vi "Modules - Test Panel.vi"(8 "error in":errorcluster) -> (0 "error out":errorcluster)   [LabVIEW 2019]
uses:
  Controls/Station - Test Type.ctl
  Controls/Test Panel - State.ctl
  Controls/eFGV States.ctl
  Controls/FGV States.ctl
  Controls/Test Panel - Data Structure.ctl
  <vilib>/Utility/miscctls.llb/LVRowAndColumnTypeDef.ctl
panel:
  in  "Add Station":bool
  in  "Test Type":T1 items=["Please Select", "Triaxial Shear", "Triaxial UU", "Shearbox", "Permeability", "Consolidation (Stepped Loading)/Swelling", "Saturation (Incremental)", "User Defined", "UCT", "Isotropic Consolidation", "Swelling Pressure"]
  in  "Data Save":bool
  out "Job Description :":string
  out "Job No :":string
  out "Sample No :":string
  in  "Add Test":bool
  in  "Sample":bool
  in  "Tab":enum32{"Test Stages"}(tab)
  out "Table":string[][](table)
  in  "Next Stage":bool caption="Go to next Stage \nautomatically"
  in  "Run":bool
  in  "Remove":bool
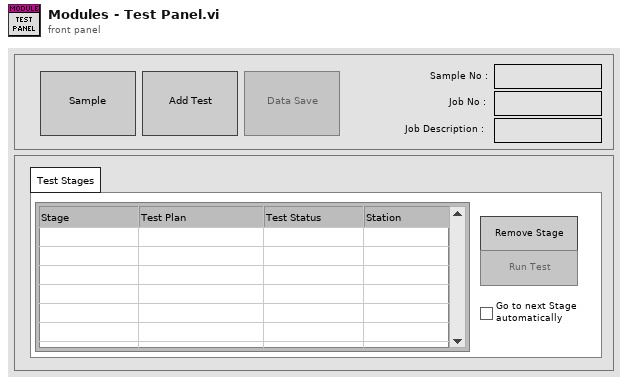
[diagram p1: front panel]
types:
  T1 = typedef "Station - Test Type.ctl" = u16
  T2 = typedef "Test Panel - State.ctl" = enum16{"Init", "Idle", "Load", "Run", "Add Test", "Highlight", "Up", "Down", "Manual", "Clear Data", "Save List", "Load List", "Change Station", "Close"}
  T3 = typedef "Test Panel - Data Structure.ctl" = cluster{"Station":string, "Sample ID":string, "Job No":string, "Job Description":string, "Filename":string, "Test Type":T1, "Speciment No":string, "Depth":string, "Height":string, "Diameter/Length":string, "Weight":string, "Test Parameter":string, "Station[]":string[], "Edit Pos":T4, "Edit Pos Prev":T4, "Area":string, "Path":string}
  T4 = typedef "LVRowAndColumnTypeDef.ctl" = cluster{"Row":i32, "Column":i32}
  T5 = enum8{"Enabled", "Disabled", "Disabled and Grayed Out"}
  T6 = typedef "FGV States.ctl" = enum16{"Read", "Write"}
  T7 = enum32{"Invalid", "Standard", "Closed", "Hidden", "Minimized", "Maximized"}
  T8 = typedef "eFGV States.ctl" = enum16{"Init", "Read", "Write", "Exit"}
  T9 = cluster{"Sample No":string, "Job No":string, "Job Desc":string, "Save":bool, "Speciment No":string, "Depth":string, "Height":string, "Diameter/Length":string, "Weight":string, "JobNo []":string[], "JobID []":string[], "JobDesc []":string[], "Speciment []":string[], "attribute":string}
  T10 = cluster{"Station Name":string, "Key Value":string[], "Key Names":string[]}[]
  T11 = cluster{"Station Name":string, "Key Value":string[], "Key Names":string[]}
  T12 = enum32{"invalid app kind", "Development System", "Run Time System", "Student Edition", "Embedded LabVIEW", "Evaluation", "Custom"}
  T13 = cluster{"TestPlan Section":string, "Key Value":string[]}[]
  T14 = cluster{"TestPlan Section":string, "Key Value":string[]}
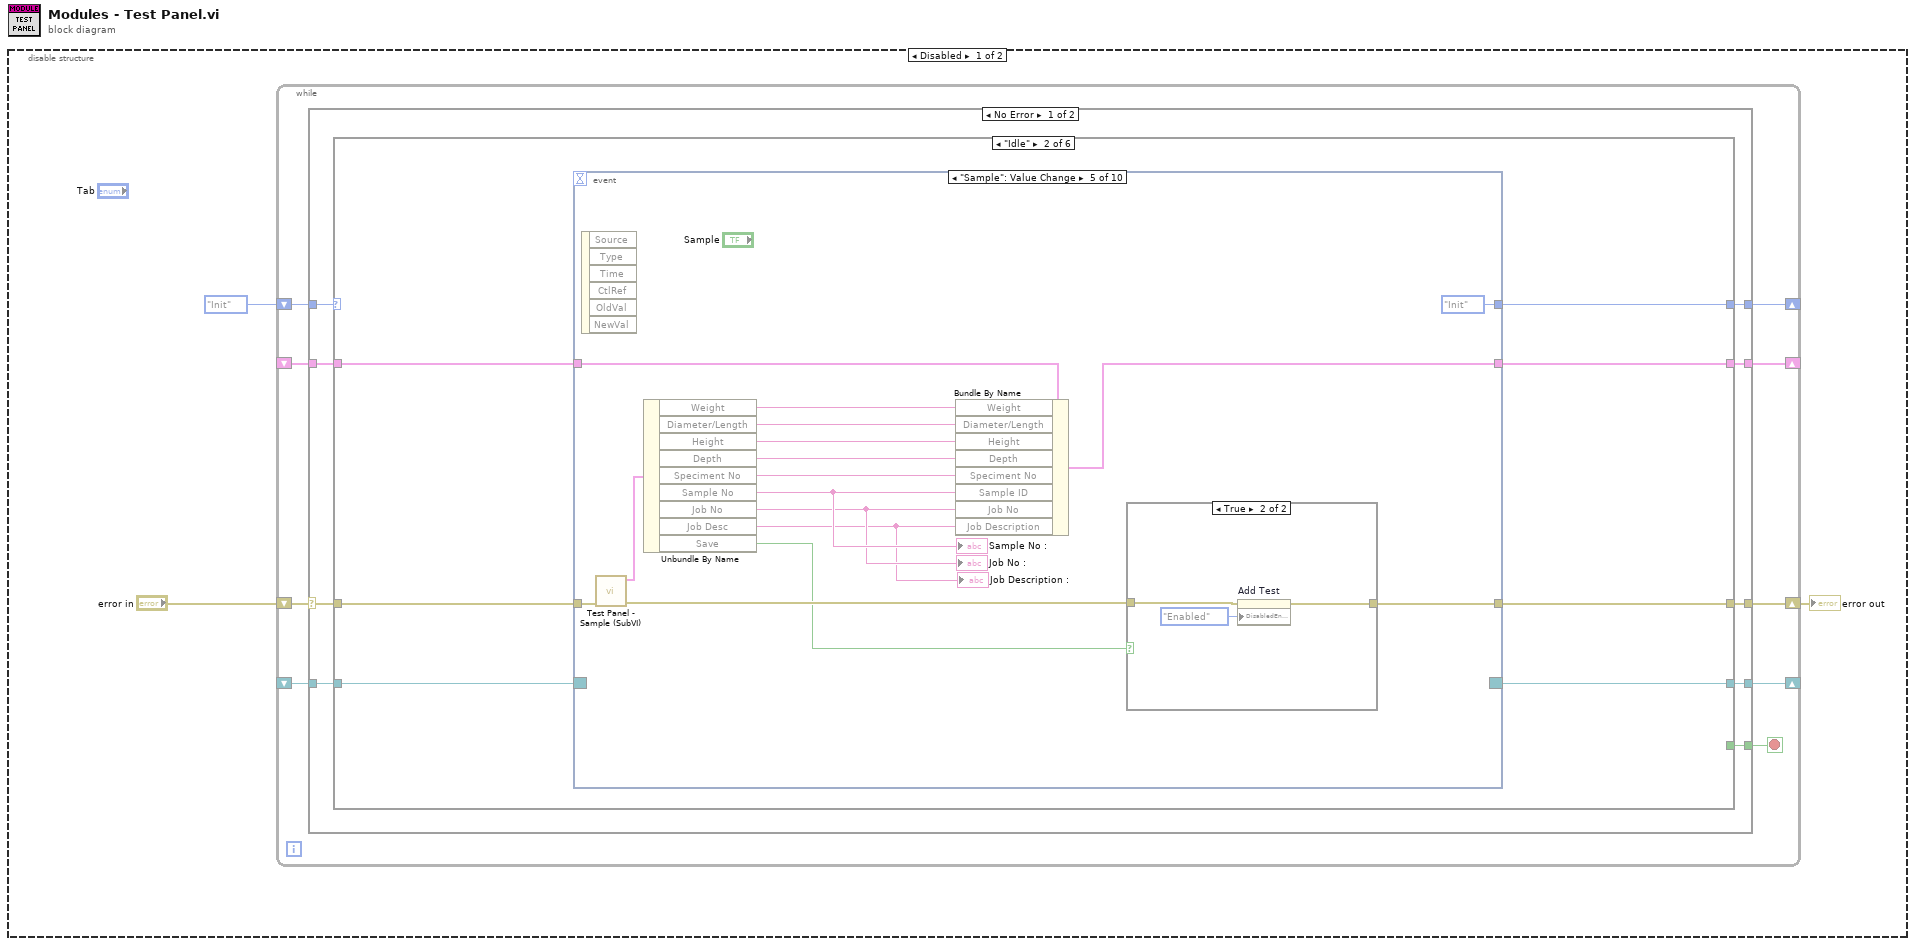
[diagram p0: block diagram]
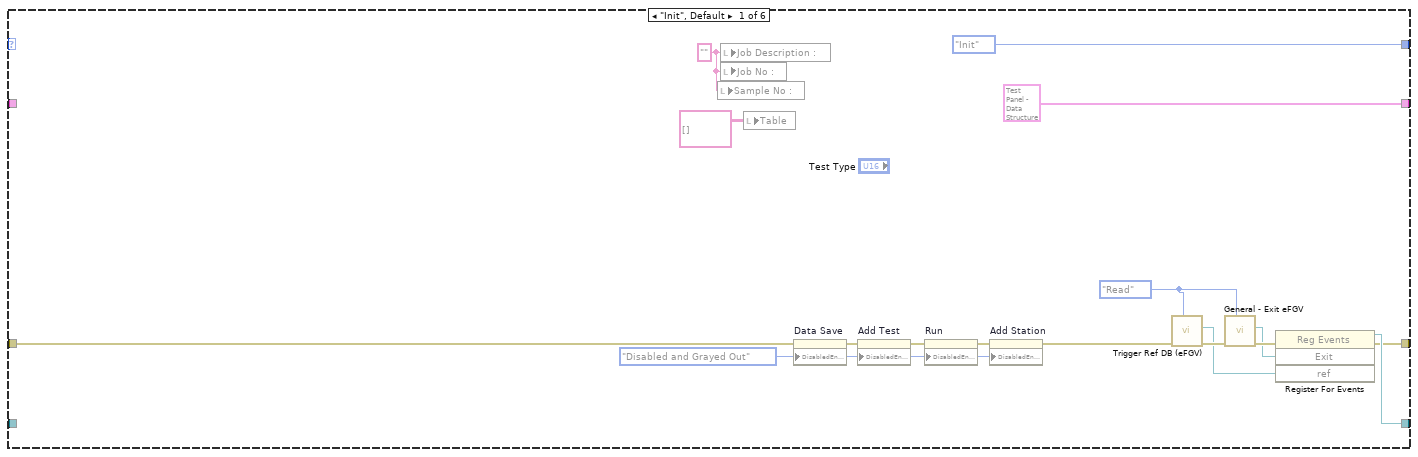
[diagram p2: hidden frame]
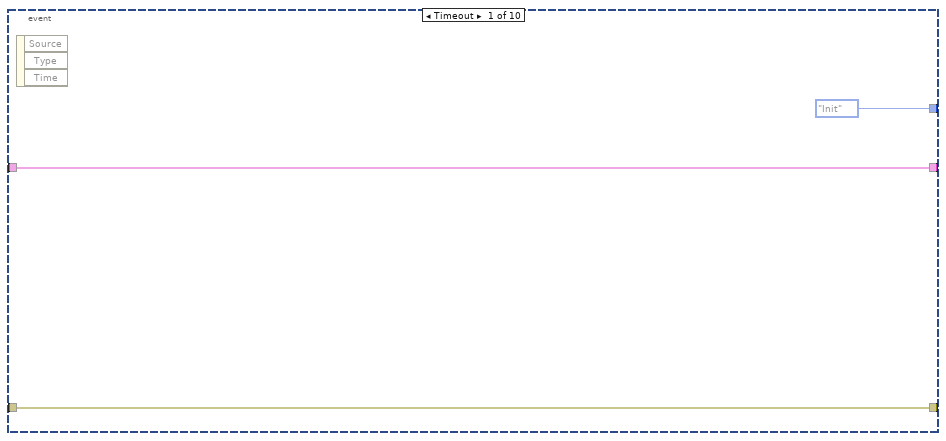
[diagram p3: hidden frame]
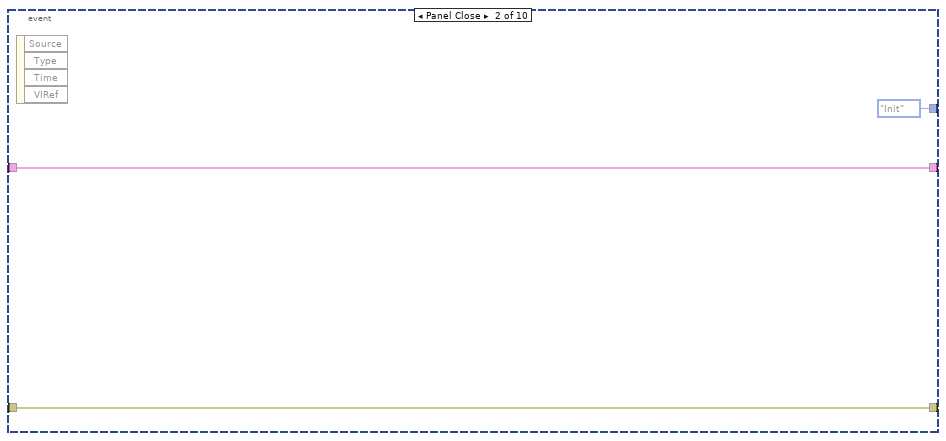
[diagram p4: hidden frame]
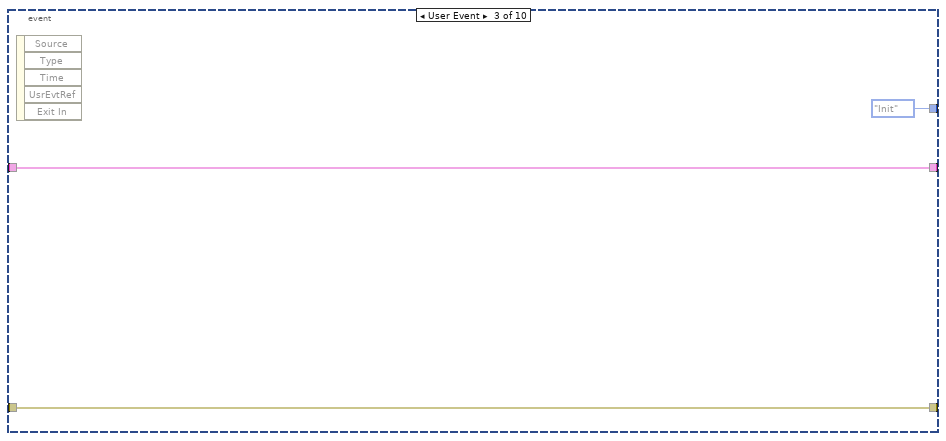
[diagram p5: hidden frame]
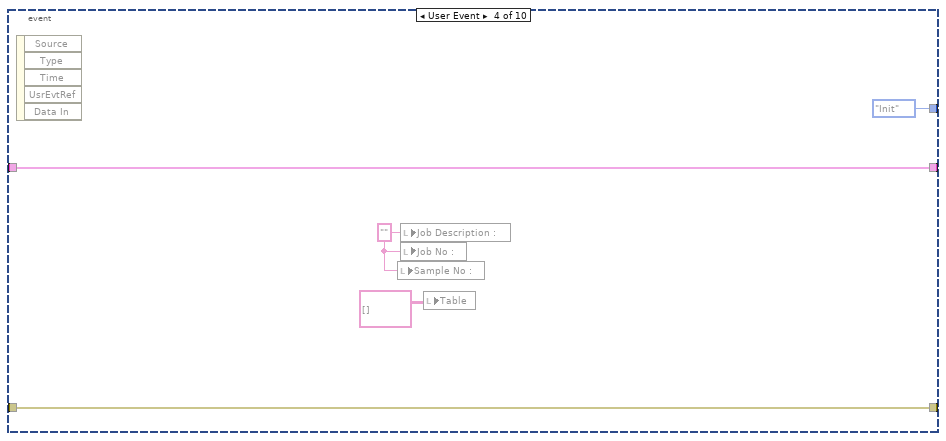
[diagram p6: hidden frame]
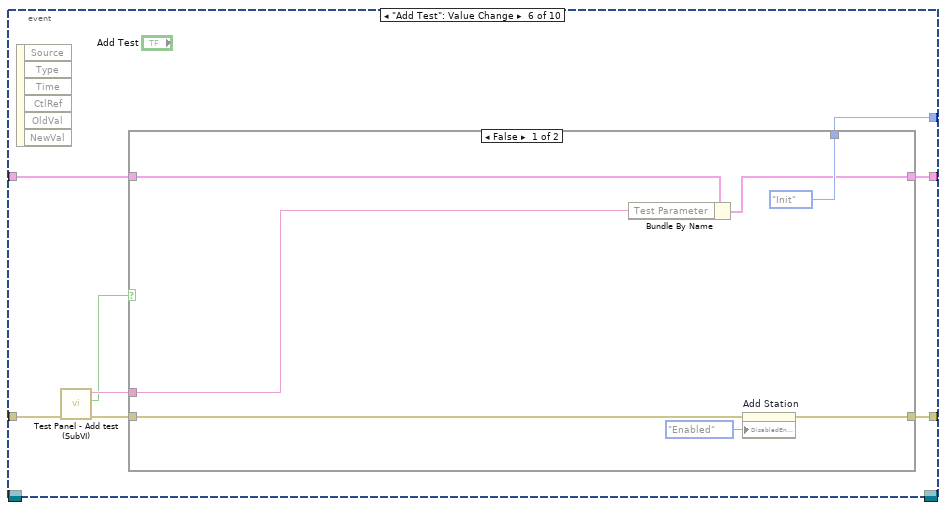
[diagram p8: hidden frame]
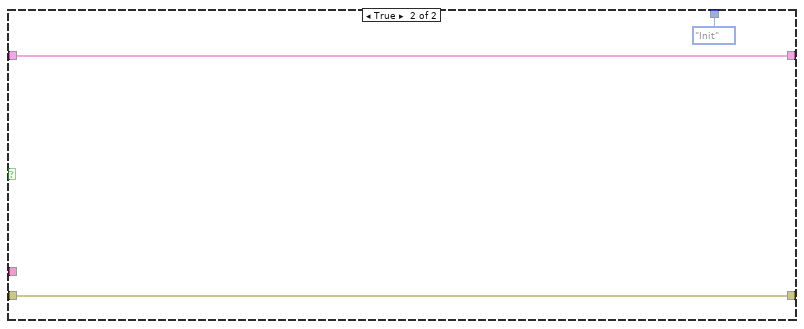
[diagram p9: hidden frame]
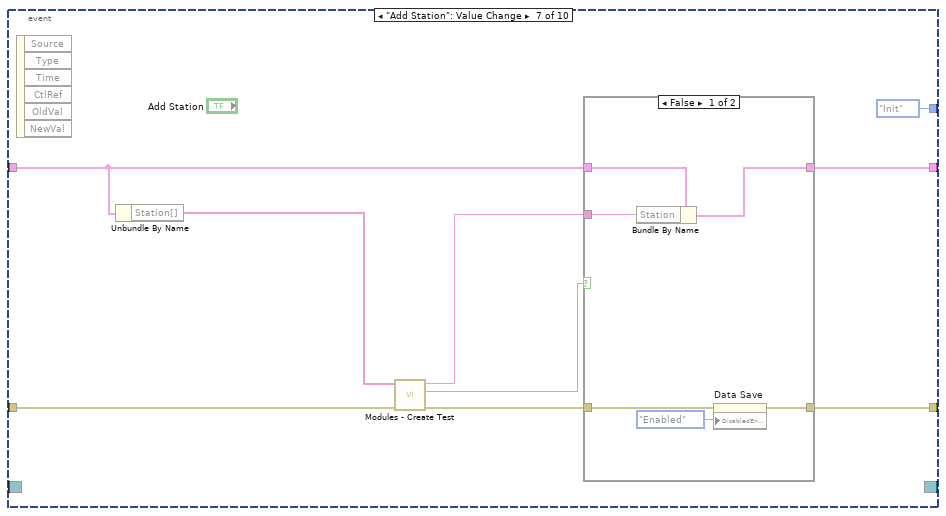
[diagram p10: hidden frame]
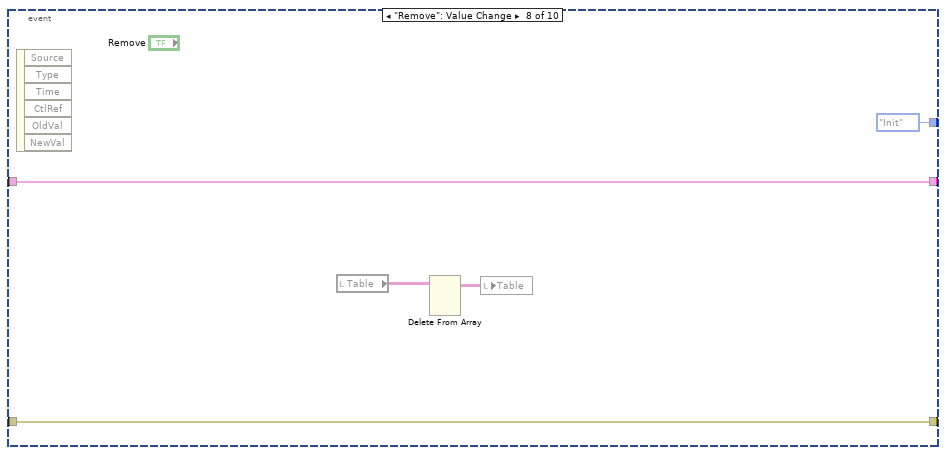
[diagram p12: hidden frame]
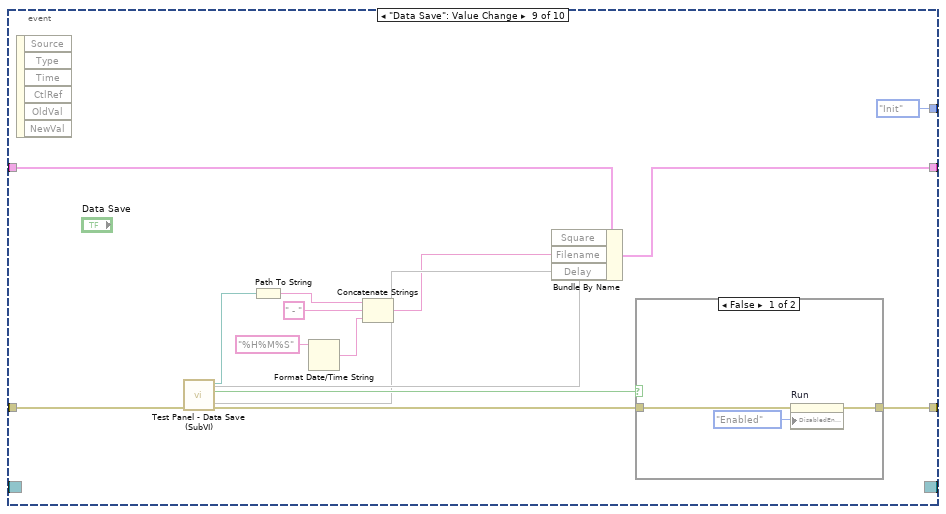
[diagram p13: hidden frame]
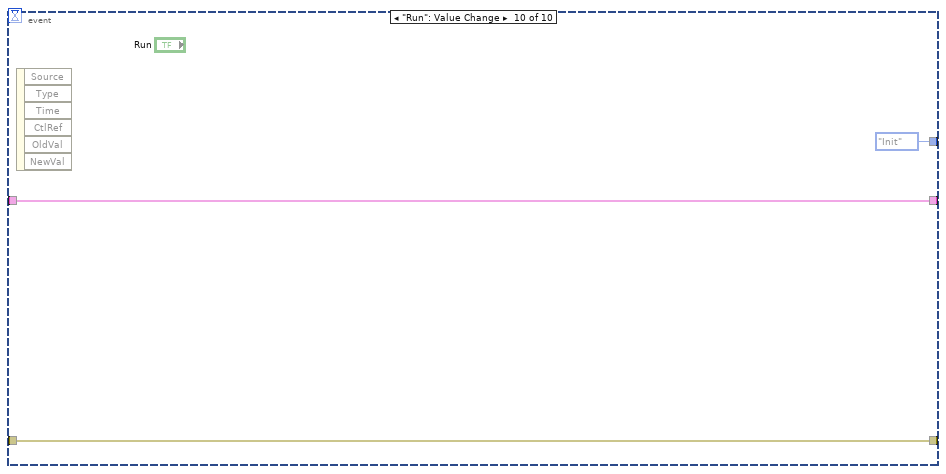
[diagram p15: hidden frame]
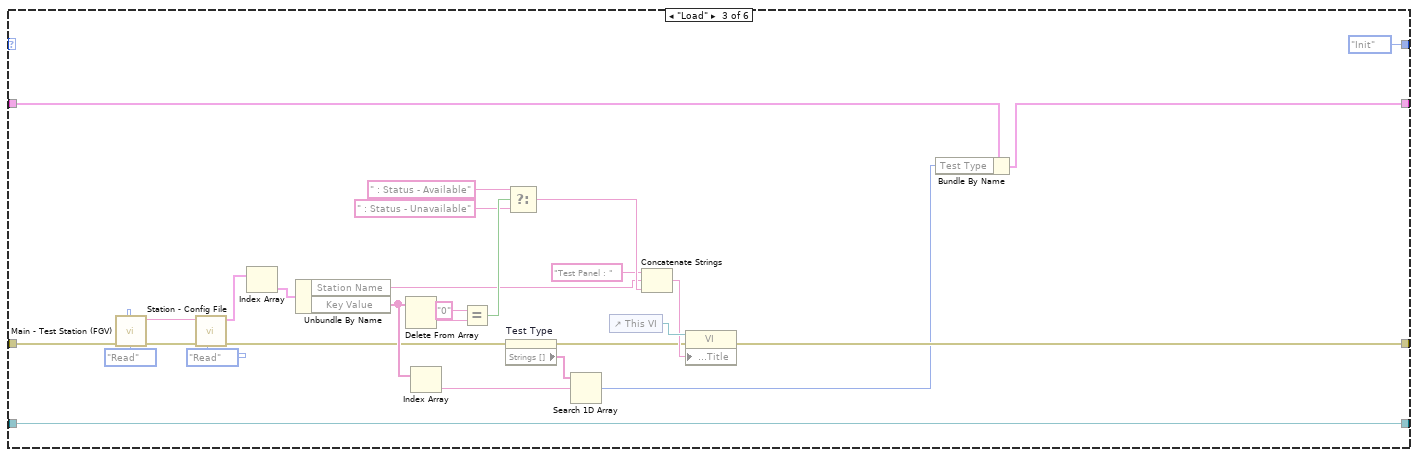
[diagram p16: hidden frame]
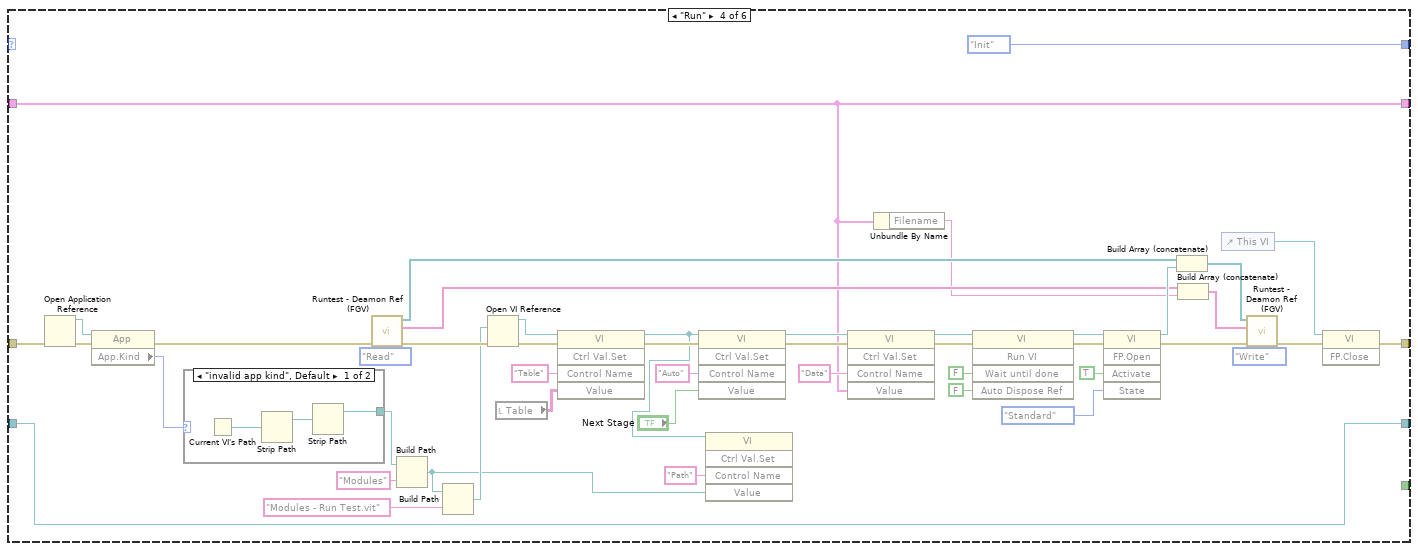
[diagram p17: hidden frame]
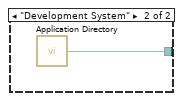
[diagram p18: hidden frame]
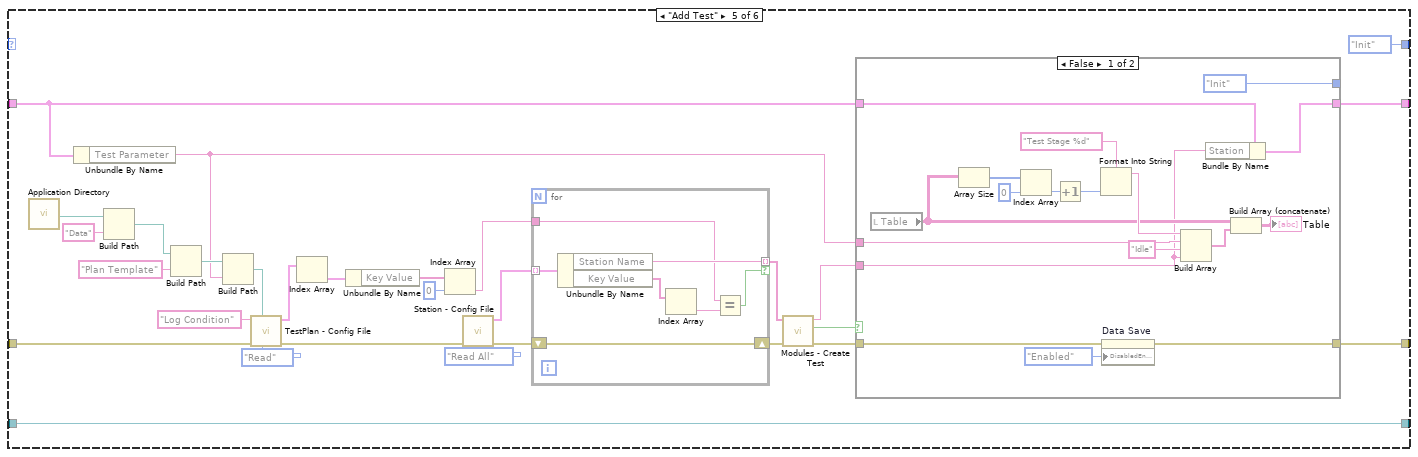
[diagram p19: hidden frame]
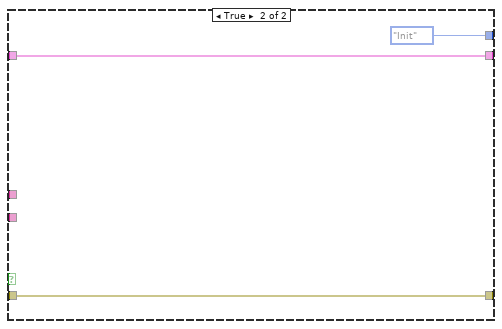
[diagram p20: hidden frame]
diagram:
  n1 = disable-structure shown="Disabled" {
    frame Disabled {
      n2 = while {
        shift-right: [w11] -> w2
        shift-left: "error in" -> [w12]
        shift-right: [w9] -> _
        shift-left: Test_Panel_-_State."Init" -> [w10]
        shift-right: [w7] -> _
        shift-left: _ -> [w6]
        shift-right: [w5] -> _
        shift-left: _ -> [w4]
        stop <- w8 stop-if-true
        n3 = case shown="No Error" w12 {
          selector: w12 -> [w20 w289]
          tunnel: [w21 w288] -> w11
          tunnel: w10 -> [w19 _]
          tunnel: [w18 Test_Panel_-_State."Init"] -> w9
          tunnel: [w17 _] -> w8
          tunnel: [w16 w285] -> w7
          tunnel: w6 -> [w15 w285]
          tunnel: [w14 w284] -> w5
          tunnel: w4 -> [w13 w284]
          frame No Error {
            n4 = case shown="\"Idle\"" w19 {
              tunnel: [w34 w45 w145 w187 w225 w278] -> w21
              tunnel: w20 -> [w29 w44 w146 w209 w236 w277]
              tunnel: [Test_Panel_-_State."Init" w43 Test_Panel_-_State."Init" Test_Panel_-_State."Init" Test_Panel_-_State."Init" Test_Panel_-_State."Init"] -> w18
              tunnel: [_ _ _ _ _ TRUE] -> w17
              tunnel: [w35 w41 w169 w208 w248 w281] -> w16
              tunnel: w15 -> [_ w42 w169 w208 w248 w281]
              tunnel: [T3 {"Station"="", "Sample ID"="", "Job No"="", "Job Description"="", "Filename"="", "Test Type"=0, "Speciment No"="", "Depth"="", "Height"="", "Diameter/Length"="", "Weight"="", "Test Parameter"="", "Station[]"=[], "Edit Pos"={"Row"=0, "Column"=0}, "Edit Pos Prev"={"Row"=0, "Column"=0}, "Area"="", "Path"=""} w40 w144 w172 w224 w280] -> w14
              tunnel: w13 -> [_ w39 w143 w172 w223 w280]
              frame "Init", Default {
                w33 = "" ("Job Description :")
                w26 = eFGV_States."Read" ("eFGV States")
                w22 = T5."Disabled and Grayed Out" ("Disabled")
                n5 = local write "Sample No :"(w33) -> ()
                n6 = local write "Job Description :"(w33) -> ()
                n7 = local write "Job No :"(w33) -> ()
                n8 = local write "Table"(string[][] []) -> ()
                n9 = property on="Data Save" class="Bool"(error in=w29, "DisabledEnum"=w22) -> (error out=w30:errorcluster)  [unwired: 1 in, 1 out]
                n10 = property on="Add Test" class="Bool"(error in=w30, "DisabledEnum"=w22) -> (error out=w31:errorcluster)  [unwired: 1 in, 1 out]
                n11 = property on="Run" class="Bool"(error in=w31, "DisabledEnum"=w22) -> (error out=w24:errorcluster)  [unwired: 1 in, 1 out]
                n12 = property on="Add Station" class="Bool"(error in=w24, "DisabledEnum"=w22) -> (error out=w23:errorcluster)  [unwired: 1 in, 1 out]
                n13 = call "Trigger Ref DB (eFGV).vi"("Action"=w26, "error in"=w23) -> ("error out"=w27:errorcluster, "ref"=w25:refnum<user-event>)  [unwired: 7 in, 1 out]
                n14 = call "General - Exit eFGV.vi"("eFGV States"=w26, "error in (no error)"=w27) -> ("error out"=w37:errorcluster, "Exit"=w36:refnum<user-event>)  [unwired: 7 in, 1 out]
                n15 = register-events(error in=w37, w36, w25) -> (reference out=w35:refnum<event-registration>, error out=w34:errorcluster)  [unwired: 1 in]
              }
              frame "Idle" {
                n16 = event shown="[4] \"Sample\": Value Change" {
                  selector: w42 -> [_ _ _ _ _ _ _ _ _ _]
                  dyn-events: [_ _ _ _ _ _ _ _ _ _] -> w41
                  timeout: _ -> [_ _ _ _ _ _ _ _ _ _]
                  tunnel: [w46 w51 w54 w59 w73 w86 w103 w119 w133 w140] -> w45
                  tunnel: w44 -> [w46 w51 w54 w59 w74 w87 w105 w119 w132 w140]
                  tunnel: [Test_Panel_-_State."Init" Test_Panel_-_State."Init" Test_Panel_-_State."Init" Test_Panel_-_State."Init" Test_Panel_-_State."Init" w80 Test_Panel_-_State."Init" Test_Panel_-_State."Init" Test_Panel_-_State."Init" Test_Panel_-_State."Init"] -> w43
                  tunnel: [w47 w50 w52 w58 w72 w82 w101 w115 w128 w139] -> w40
                  tunnel: w39 -> [w47 w50 w52 w58 w71 w83 w99 w115 w129 w139]
                  event Timeout {
                    n17 = event-data() -> ()  [unwired: 1 in, 3 out]
                  }
                  event Panel Close {
                    n18 = event-data() -> ()  [unwired: 1 in, 4 out]
                  }
                  event User Event {
                    n19 = event-data() -> ()  [unwired: 1 in, 5 out]
                  }
                  event User Event {
                    w55 = "" ("Job Description :")
                    n20 = event-data() -> ()  [unwired: 1 in, 5 out]
                    n21 = local write "Sample No :"(w55) -> ()
                    n22 = local write "Job Description :"(w55) -> ()
                    n23 = local write "Job No :"(w55) -> ()
                    n24 = local write "Table"(string[][] []) -> ()
                  }
                  event "Sample": Value Change {
                    n25 = event-data() -> ()  [unwired: 1 in, 6 out]
                    n26 = call "Test Panel - Sample (SubVI).vi"("error in"=w74) -> ("error out"=w70:errorcluster, "Data Out"=w69:T9)  [unwired: 9 in]
                    n27 = Unbundle By Name(w69) -> ("Weight"=w60:string, "Diameter/Length"=w61:string, "Height"=w62:string, "Depth"=w63:string, "Speciment No"=w64:string, "Sample No"=w68:string, "Job No"=w67:string, "Job Desc"=w66:string, "Save"=w65:bool)
                    "Sample No :" <- w68
                    "Job No :" <- w67
                    "Job Description :" <- w66
                    n28 = Bundle By Name(cluster=w71, "Weight"=w60, "Diameter/Length"=w61, "Height"=w62, "Depth"=w63, "Speciment No"=w64, "Sample ID"=w68, "Job No"=w67, "Job Description"=w66) -> (w72:T3)
                    n29 = case shown="True" w65 {
                      tunnel: [w76 w79] -> w73
                      tunnel: w70 -> [w76 w77]
                      frame False {
                      }
                      frame True {
                        n30 = property on="Add Test" class="Bool"(error in=w77, "DisabledEnum"=T5."Enabled" ("Disabled")) -> (error out=w79:errorcluster)  [unwired: 1 in, 1 out]
                      }
                    }
                  }
                  event "Add Test": Value Change {
                    n31 = event-data() -> ()  [unwired: 1 in, 6 out]
                    n32 = call "Test Panel - Add test (SubVI).vi"("error in"=w87) -> ("error Out"=w84:errorcluster, "Cancel?"=w81:bool, "Test Plan"=w85:string)  [unwired: 6 in, 2 out]
                    n33 = case shown="False" w81 {
                      tunnel: [w94 w96] -> w86
                      tunnel: w85 -> [w88 _]
                      tunnel: w84 -> [w93 w96]
                      tunnel: w83 -> [w89 w97]
                      tunnel: [w90 w97] -> w82
                      tunnel: [Test_Panel_-_State."Init" Test_Panel_-_State."Init"] -> w80
                      frame False {
                        n34 = Bundle By Name(cluster=w89, "Test Parameter"=w88) -> (w90:T3)
                        n35 = property on="Add Station" class="Bool"(error in=w93, "DisabledEnum"=T5."Enabled" ("Disabled")) -> (error out=w94:errorcluster)  [unwired: 1 in, 1 out]
                      }
                      frame True {
                      }
                    }
                  }
                  event "Add Station": Value Change {
                    n36 = event-data() -> ()  [unwired: 1 in, 6 out]
                    n37 = Unbundle By Name(w99) -> ("Station[]"=w98:string[])
                    n38 = call "Modules - Create Test.vi"("error in"=w105, "Station"=w98) -> ("error out"=w104:errorcluster, "Cancel out"=w100:bool, "Stations"=w102:string)  [unwired: 7 in]
                    n39 = case shown="False" w100 {
                      tunnel: w104 -> [w111 w113]
                      tunnel: [w110 w113] -> w103
                      tunnel: w102 -> [w109 _]
                      tunnel: [w108 w114] -> w101
                      tunnel: w99 -> [w107 w114]
                      frame False {
                        n40 = Bundle By Name(cluster=w107, "Station"=w109) -> (w108:T3)
                        n41 = property on="Data Save" class="Bool"(error in=w111, "DisabledEnum"=T5."Enabled" ("Disabled")) -> (error out=w110:errorcluster)  [unwired: 1 in, 1 out]
                      }
                      frame True {
                      }
                    }
                  }
                  event "Remove": Value Change {
                    n42 = event-data() -> ()  [unwired: 1 in, 6 out]
                    n43 = local read "Table"() -> (w117:string[][])
                    n44 = Delete From Array(array=w117) -> (array with subset deleted=w116:string[][])  [unwired: 3 in, 1 out]
                    n45 = local write "Table"(w116) -> ()
                  }
                  event "Data Save": Value Change {
                    n46 = event-data() -> ()  [unwired: 1 in, 6 out]
                    n47 = call "Test Panel - Data Save (SubVI).vi"("error in"=w132) -> ("error Out"=w131:errorcluster, "Cancel?"=w130:bool, "Select Report Path out"=w121:path, 4:w126, 5:w127)  [unwired: 6 in]
                    n48 = Path To String(path=w121) -> (string=w124:string)
                    n49 = Format Date/Time String(time format string (%c)="%H%M%S") -> (date/time string=w122:string)  [unwired: 2 in]
                    n50 = Concatenate Strings(w124, " - " ("string"), w122) -> (w120:string)
                    n51 = Bundle By Name(cluster=w129, "Square"=w127, "Filename"=w120, "Delay"=w126) -> (w128:T3)
                    n52 = case shown="False" w130 {
                      tunnel: [w136 w138] -> w133
                      tunnel: w131 -> [w135 w138]
                      frame False {
                        n53 = property on="Run" class="Bool"(error in=w135, "DisabledEnum"=T5."Enabled" ("Disabled")) -> (error out=w136:errorcluster)  [unwired: 1 in, 1 out]
                      }
                      frame True {
                      }
                    }
                  }
                  event "Run": Value Change {
                    n54 = event-data() -> ()  [unwired: 1 in, 6 out]
                  }
                }
              }
              frame "Load" {
                n55 = call "Main - Test Station (FGV).vi"("Action"=FGV_States."Read", "error In"=w146) -> ("error out"=w164:errorcluster, "Station Name out"=w165:string)  [unwired: 8 in]
                n56 = call "Station - Config File.vi"("Action"=enum16{"Write", "Read", "Read All", "Remove"}."Read", "error in (no error)"=w164, "Station Name"=w165) -> ("error out"=w156:errorcluster, "Value Out"=w163:T10)  [unwired: 7 in]
                n57 = Index Array(array=w163) -> (element=w162:T11)  [unwired: 1 in]
                n58 = Unbundle By Name(w162) -> ("Station Name"=w158:string, "Key Value"=w157:string[])
                n59 = Delete From Array(array=w157) -> (deleted portion=w161:string)  [unwired: 2 in, 1 out]
                n60 = Index Array(array=w157) -> (element=w153:string)  [unwired: 1 in]
                n61 = Equal?(x="0", y=w161) -> (x = y?=w160:bool)
                n62 = property on="Test Type" class="Ring (strict)"(error in=w156) -> (error out=w155:errorcluster, "Strings []"=w154:string[])  [unwired: 1 in, 1 out]
                n63 = Select(t=" : Status - Available" ("string"), s=w160, f=" : Status - Unavailable" ("string")) -> (s? t:f=w159:string)
                n64 = Search 1D Array(1D array=w154, element=w153) -> (index of element=w142:i32)  [unwired: 1 in]
                n65 = control-ref of="This VI"() -> (w167:refnum<vi>)
                n66 = Concatenate Strings("Test Panel : " ("string"), w158, w159) -> (w166:string)
                n67 = property class="VI"(reference=w167, error in=w155, "Front Panel.Title"=w166) -> (error out=w145:errorcluster)  [unwired: 1 out]
                n68 = Bundle By Name(cluster=w143, "Test Type"=w142) -> (w144:T3)
              }
              frame "Run" {
                n69 = Open Application Reference(8:w209) -> (0:w213:errorcluster, 3:w212:refnum<vi>)  [unwired: 3 in]
                n70 = property class="App"(reference=w212, error in=w213) -> (error out=w186:errorcluster, "App.Kind"=w211:T12)  [unwired: 1 out]
                n71 = case shown="\"invalid app kind\", Default" w211 {
                  tunnel: [w216 w219] -> w210
                  frame "invalid app kind", Default {
                    n72 = Current VI's Path() -> (path=w218:path)
                    n73 = Strip Path(path=w218) -> (stripped path=w217:path)  [unwired: 1 out]
                    n74 = Strip Path(path=w217) -> (stripped path=w216:path)  [unwired: 1 out]
                  }
                  frame "Development System" {
                    n75 = call <vilib>:"Application Directory.vi"() -> ("Application Directory"=w219:path)
                  }
                }
                n76 = call "Runtest - Deamon Ref (FGV).vi"("Action"=FGV_States."Read", "error in"=w186) -> ("error out"=w185:errorcluster, "Name out"=w173:string[], "Ref out"=w182:refnum<vi>[])  [unwired: 7 in]
                n77 = Build Path(base path=w210, name or relative path="Modules") -> (appended path=w174:path)
                n78 = Build Path(base path=w174, name or relative path="Modules - Run Test.vit") -> (appended path=w175:path)
                n79 = Open VI Reference(vi path=w175, error in (no error)=w185) -> (vi reference=w197:refnum<vi>, error out=w198:errorcluster)  [unwired: 4 in]
                n80 = local read "Table"() -> (w206:string[][])
                n81 = invoke class="VI" method="Ctrl Val.Set"(reference=w197, error in=w198, "Control Name"="Table", "Value"=w206) -> (reference out=w177:refnum<vi>, error out=w203:errorcluster)  [unwired: 1 in, 3 out]
                n82 = invoke class="VI" method="Ctrl Val.Set"(reference=w177, error in=w203, "Control Name"="Auto", "Value"="Next Stage") -> (reference out=w200:refnum<vi>, error out=w199:errorcluster)  [unwired: 1 in, 3 out]
                n83 = invoke class="VI" method="Ctrl Val.Set"(reference=w177, "Control Name"="Path", "Value"=w174) -> ()  [unwired: 2 in, 5 out]
                n84 = invoke class="VI" method="Ctrl Val.Set"(reference=w200, error in=w199, "Control Name"="Data", "Value"=w172) -> (reference out=w189:refnum<vi>, error out=w190:errorcluster)  [unwired: 1 in, 3 out]
                n85 = Unbundle By Name(w172) -> ("Filename"=w171:string)
                n86 = invoke class="VI" method="Run VI"(reference=w189, error in=w190, "Wait until done"=FALSE ("Wait Until Done"), "Auto Dispose Ref"=FALSE ("Auto Dispose Reference")) -> (reference out=w194:refnum<vi>, error out=w193:errorcluster)  [unwired: 1 in, 3 out]
                n87 = invoke class="VI" method="FP.Open"(reference=w194, error in=w193, "Activate"=TRUE ("Activate?"), "State"=T7."Standard") -> (reference out=w183:refnum<vi>, error out=w180:errorcluster)  [unwired: 1 in, 3 out]
                n88 = Build Array (concatenate)(w182, w183) -> (w178:refnum<vi>[])
                n89 = Build Array (concatenate)(w173, w171) -> (w170:string[])
                n90 = control-ref of="This VI"() -> (w188:refnum<vi>)
                n91 = call "Runtest - Deamon Ref (FGV).vi"("Action"=FGV_States."Write", "error in"=w180, "Name"=w170, "Ref in"=w178) -> ("error out"=w179:errorcluster)  [unwired: 5 in, 2 out]
                n92 = invoke class="VI" method="FP.Close"(reference=w188, error in=w179) -> (error out=w187:errorcluster)  [unwired: 1 in, 2 out]
              }
              frame "Add Test" {
                n93 = call <vilib>:"Application Directory.vi"() -> ("Application Directory"=w242:path)
                n94 = Unbundle By Name(w223) -> ("Test Parameter"=w222:string)
                n95 = Build Path(base path=w242, name or relative path="Data") -> (appended path=w243:path)
                n96 = Build Path(base path=w243, name or relative path="Plan Template") -> (appended path=w241:path)
                n97 = Build Path(base path=w241, name or relative path=w222) -> (appended path=w246:path)
                n98 = call "TestPlan - Config File.vi"("Action"=enum16{"Write", "Read", "Read All", "Remove"}."Read", "file path"=w246, "error in (no error)"=w236, "TestPlan Section"="Log Condition") -> ("error out"=w232:errorcluster, "Value Out"=w244:T13)  [unwired: 5 in, 1 out]
                n99 = Index Array(array=w244) -> (element=w245:T14)  [unwired: 1 in]
                n100 = Unbundle By Name(w245) -> ("Key Value"=w235:string[])
                n101 = Index Array(array=w235, index=0) -> (element=w229:string)
                n102 = call "Station - Config File.vi"("Action"=enum16{"Write", "Read", "Read All", "Remove"}."Read All", "error in (no error)"=w232) -> ("error out"=w230:errorcluster, "Value Out"=w231:T10)  [unwired: 8 in]
                n103 = for {
                  tunnel: w231 -> [w276] mode=indexing
                  tunnel: [w274] -> w228 mode=indexing if=w270
                  tunnel: w229 -> [w271]
                  shift-right: [w273] -> w227
                  shift-left: w230 -> [w273]
                  n104 = Unbundle By Name(w276) -> ("Station Name"=w274:string, "Key Value"=w275:string[])
                  n105 = Index Array(array=w275) -> (element=w272:string)  [unwired: 1 in]
                  n106 = Equal?(x=w271, y=w272) -> (x = y?=w270:bool)
                }
                n107 = call "Modules - Create Test.vi"("error in"=w227, "Station"=w228) -> ("error out"=w226:errorcluster, "Cancel out"=w220:bool, "Stations"=w221:string)  [unwired: 7 in]
                n108 = case shown="False" w220 {
                  tunnel: [w257 w268] -> w225
                  tunnel: w222 -> [w253 _]
                  tunnel: w226 -> [w256 w268]
                  tunnel: w223 -> [w249 w269]
                  tunnel: [w250 w269] -> w224
                  tunnel: [Test_Panel_-_State."Init" Test_Panel_-_State."Init"] -> _
                  tunnel: w221 -> [w251 _]
                  frame False {
                    n109 = local read "Table"() -> (w259:string[][])
                    n110 = Array Size(array=w259) -> (size(s)=w266:i32[])
                    n111 = Index Array(array=w266, index=0) -> (element=w264:i32)
                    n112 = Increment(x=w264) -> (x+1=w262:i32)
                    n113 = Format Into String(format string="Test Stage %d", w262) -> (resulting string=w261:string)  [unwired: 2 in, 1 out]
                    n114 = property on="Data Save" class="Bool"(error in=w256, "DisabledEnum"=T5."Enabled" ("Disabled")) -> (error out=w257:errorcluster)  [unwired: 1 in, 1 out]
                    n115 = Build Array(w261, w253, "Idle" ("element"), w251) -> (w258:string[])
                    n116 = Bundle By Name(cluster=w249, "Station"=w251) -> (w250:T3)
                    n117 = Build Array (concatenate)(w259, w258) -> (→"Table":string[][])
                  }
                  frame True {
                  }
                }
              }
              frame "Close" {
                n118 = control-ref of="This VI"() -> (w279:refnum<vi>)
                n119 = invoke class="VI" method="FP.Close"(reference=w279, error in=w277) -> (error out=w278:errorcluster)  [unwired: 1 in, 2 out]
              }
            }
          }
          frame Error {
            n120 = call <vilib>:"Clear Errors.vi"("error in (no error)"=w289) -> ("error out"=w288:errorcluster)  [unwired: 5 in, 1 out]
            n121 = Wait (ms)(milliseconds to wait=u32 100) -> ()  [unwired: 1 out]
          }
        }
      }
      "error out" <- w2
    }
    frame Enabled {
    }
  }
